vi "Convert Buttons.vi"(7 "POVs":i16[](array[numeric]), 8 "HW_Button Board":bool[](array[boolean]), 9 "HW_Button Board_Axes":dbl[](array[numeric]), 10 "HW_Joystick_Buttons":bool[](array[boolean]), 11 "HW_Joystick_Axes":dbl[](array[numeric])) -> ()   [LabVIEW 2017, in "Controller.lvlib"]
doc: "This VI provides a central place to assign joystick buttons to sepcifc tasks. It aids in the readability of the code and makes it easier to change button assignments."
uses:
  Controller.lvlib
  ENUM_Botton Board.ctl
  ENUM_Logitech Extrem 3D Pro Buttons.ctl
  Global Control Outputs.vi
  ENUM_Logitech GamePad Button List.ctl
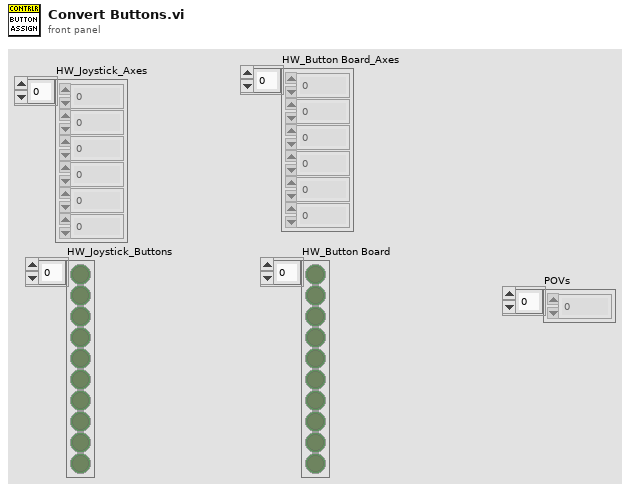
[diagram p1: front panel]
types:
  T1 = typedef "Controller.lvlib/ENUM_Botton Board.ctl" = enum16{"Top Right", "Top Left", "Center Right", "Center Middle", "Center Left", "Bottom Right", "Bottom Middle", "Botton Left"}
  T2 = typedef "Controller.lvlib/ENUM_Logitech GamePad Button List.ctl" = enum16{"Right Pad A-Green", "Right Pad B-Red", "Right Pad X-Blue", "Right Pad Y-Yellow", "Left Trigger LB", "Right Trigger RB", "Center Pad Back", "Center Pad Start", "Left Thumb", "Right Thumb"}
  T3 = typedef "Controller.lvlib/ENUM_Logitech Extrem 3D Pro Buttons.ctl" = enum16{"Trigger (1)", "Thumb (2)", "Upper Top Left (5)", "Upper Lower Left (3)", "Upper Top Right (6)", "Upper Lower Right (4)", "Lower Front Left (7)", "Lower Front Right (8)", "Lower Middle Left (9)", "Lower Middle Right (10)", "Lower Back Left (11)", "Lower (Back Right (12)"}
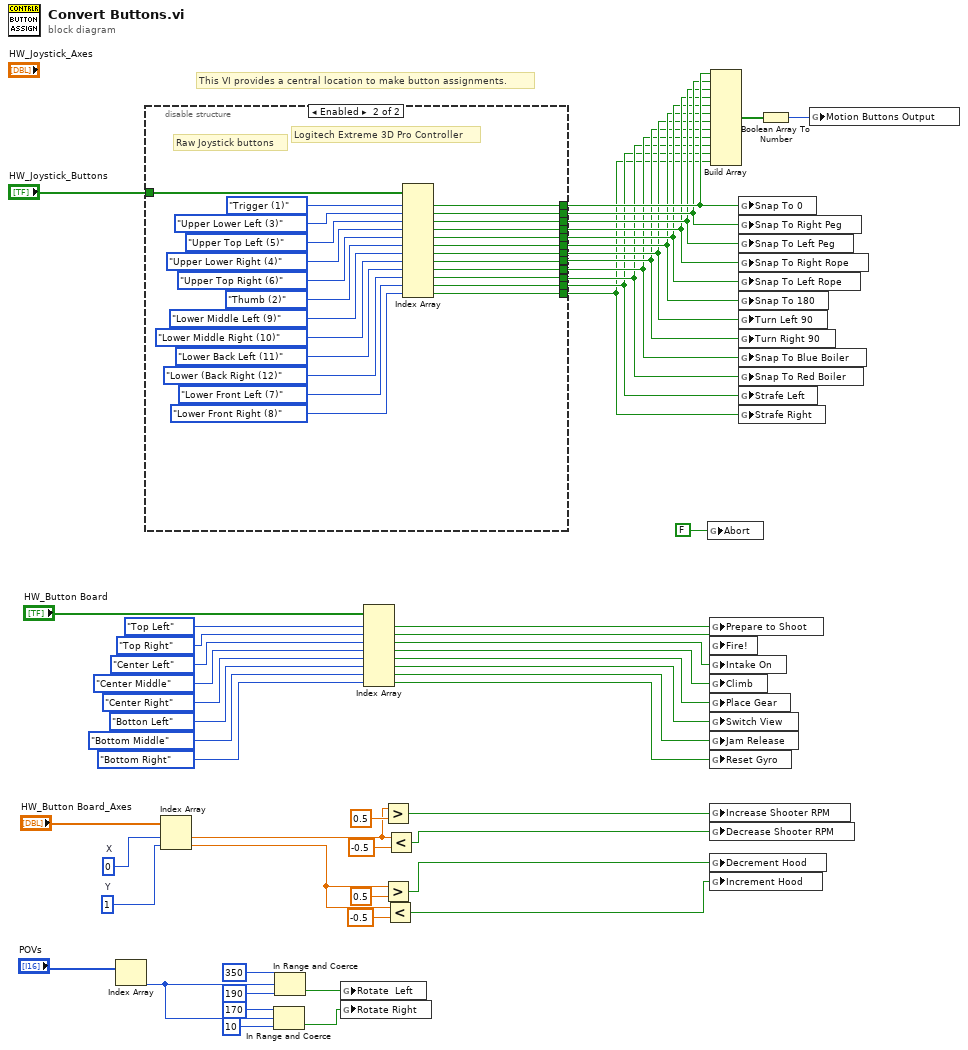
[diagram p0: block diagram]
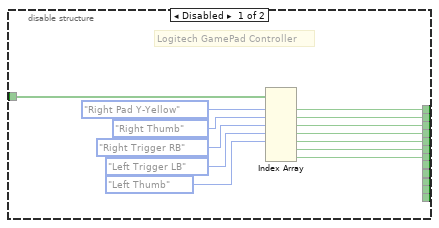
[diagram p2: hidden frame]
diagram:
  w19 = 1  # Y
  w20 = 0  # X
  # "This VI provides a central location to make button assignments."
  n1 = Index Array(array="POVs") -> (element=w7:i16)  [unwired: 1 in]
  n2 = disable-structure shown="Enabled" {
    disable-tunnel: "HW_Joystick_Buttons" -> [w67 w92]
    disable-tunnel: [w65 w87] -> w52
    disable-tunnel: [w61 w86] -> w51
    disable-tunnel: [w60 w85] -> w50
    disable-tunnel: [w59 w84] -> w49
    disable-tunnel: [w57 w82] -> w47
    disable-tunnel: [w56 w81] -> w46
    disable-tunnel: [w55 w83] -> w48
    disable-tunnel: [_ w80] -> w45
    disable-tunnel: [_ w79] -> w44
    disable-tunnel: [_ w78] -> w43
    disable-tunnel: [_ w77] -> w42
    disable-tunnel: [_ w76] -> w41
    frame Disabled {
      # "Logitech GamePad Controller"
      n3 = Index Array(array=w67, index #1=ENUM_Logitech_GamePad_Button_List."Right Pad Y-Yellow" ("Controler Button List"), index #2=ENUM_Logitech_GamePad_Button_List."Right Thumb" ("Controler Button List"), index #3=ENUM_Logitech_GamePad_Button_List."Right Trigger RB" ("Controler Button List"), index #4=ENUM_Logitech_GamePad_Button_List."Left Trigger LB" ("Controler Button List"), index #5=ENUM_Logitech_GamePad_Button_List."Left Thumb" ("Controler Button List")) -> (element #1=w65:bool, element #2=w61:bool, element #3=w60:bool, element #4=w59:bool, element #5=w55:bool, element #6=w57:bool, element #7=w56:bool)  [unwired: 2 in]
    }
    frame Enabled {
      # "Raw Joystick buttons"
      # "Logitech Extreme 3D Pro Controller"
      n4 = Index Array(array=w92, index #1=ENUM_Logitech_Extrem_3D_Pro_Buttons."Trigger (1)" ("Logitech Extreme 3D Pro Buttons"), index #2=ENUM_Logitech_Extrem_3D_Pro_Buttons."Upper Lower Left (3)" ("Logitech Extreme 3D Pro Buttons"), index #3=ENUM_Logitech_Extrem_3D_Pro_Buttons."Upper Top Left (5)" ("Logitech Extreme 3D Pro Buttons"), index #4=ENUM_Logitech_Extrem_3D_Pro_Buttons."Upper Lower Right (4)" ("Logitech Extreme 3D Pro Buttons"), index #5=ENUM_Logitech_Extrem_3D_Pro_Buttons."Upper Top Right (6)" ("Logitech Extreme 3D Pro Buttons"), index #6=ENUM_Logitech_Extrem_3D_Pro_Buttons."Thumb (2)" ("Logitech Extreme 3D Pro Buttons"), index #7=ENUM_Logitech_Extrem_3D_Pro_Buttons."Lower Middle Left (9)" ("Logitech Extreme 3D Pro Buttons"), index #8=ENUM_Logitech_Extrem_3D_Pro_Buttons."Lower Middle Right (10)" ("Logitech Extreme 3D Pro Buttons"), index #9=ENUM_Logitech_Extrem_3D_Pro_Buttons."Lower Back Left (11)" ("Logitech Extreme 3D Pro Buttons"), index #10=ENUM_Logitech_Extrem_3D_Pro_Buttons."Lower (Back Right (12)" ("Logitech Extreme 3D Pro Buttons"), index #11=ENUM_Logitech_Extrem_3D_Pro_Buttons."Lower Front Left (7)" ("Logitech Extreme 3D Pro Buttons"), index #12=ENUM_Logitech_Extrem_3D_Pro_Buttons."Lower Front Right (8)" ("Logitech Extreme 3D Pro Buttons")) -> (element #1=w87:bool, element #2=w86:bool, element #3=w85:bool, element #4=w84:bool, element #5=w83:bool, element #6=w82:bool, element #7=w81:bool, element #8=w80:bool, element #9=w79:bool, element #10=w78:bool, element #11=w77:bool, element #12=w76:bool)
    }
  }
  n5 = Index Array(array="HW_Button Board_Axes", index #1=w20, index #2=w19) -> (element #1=w15:dbl, element #2=w9:dbl)
  n6 = In Range and Coerce(upper limit=i16 170, x=w7, lower limit=i16 10) -> (In Range?=w1:bool)  [unwired: 1 out]
  n7 = In Range and Coerce(upper limit=i16 350, x=w7, lower limit=i16 190) -> (In Range?=w2:bool)  [unwired: 1 out]
  n8 = global write "Global Control Outputs.vi" "Rotate  Left"(w2) -> ()
  n9 = global write "Global Control Outputs.vi" "Rotate Right"(w1) -> ()
  n10 = Index Array(array="HW_Button Board", index #1=ENUM_Botton_Board."Top Left" ("Control Board Buttons"), index #2=ENUM_Botton_Board."Top Right" ("Control Board Buttons"), index #3=ENUM_Botton_Board."Center Left" ("Control Board Buttons"), index #4=ENUM_Botton_Board."Center Middle" ("Control Board Buttons"), index #5=ENUM_Botton_Board."Center Right" ("Control Board Buttons"), index #6=ENUM_Botton_Board."Botton Left" ("Control Board Buttons"), index #7=ENUM_Botton_Board."Bottom Middle" ("Control Board Buttons"), index #8=ENUM_Botton_Board."Bottom Right" ("Control Board Buttons")) -> (element #1=w39:bool, element #2=w30:bool, element #3=w29:bool, element #4=w28:bool, element #5=w27:bool, element #6=w26:bool, element #7=w25:bool, element #8=w24:bool)
  n11 = Greater?(x=w15, y=0.5) -> (0:w17:bool)
  n12 = Greater?(x=w9, y=0.5) -> (0:w12:bool)
  n13 = Less?(x=w9, y=-0.5) -> (x < y?=w13:bool)
  n14 = Less?(x=w15, y=-0.5) -> (x < y?=w14:bool)
  n15 = global write "Global Control Outputs.vi" "Abort"(FALSE) -> ()
  n16 = global write "Global Control Outputs.vi" "Prepare to Shoot"(w39) -> ()
  n17 = global write "Global Control Outputs.vi" "Fire!"(w30) -> ()
  n18 = global write "Global Control Outputs.vi" "Intake On"(w29) -> ()
  n19 = global write "Global Control Outputs.vi" "Climb"(w28) -> ()
  n20 = global write "Global Control Outputs.vi" "Place Gear"(w27) -> ()
  n21 = global write "Global Control Outputs.vi" "Switch View"(w26) -> ()
  n22 = global write "Global Control Outputs.vi" "Jam Release"(w25) -> ()
  n23 = global write "Global Control Outputs.vi" "Reset Gyro"(w24) -> ()
  n24 = global write "Global Control Outputs.vi" "Increase Shooter RPM"(w17) -> ()
  n25 = global write "Global Control Outputs.vi" "Decrease Shooter RPM"(w14) -> ()
  n26 = global write "Global Control Outputs.vi" "Decrement Hood"(w12) -> ()
  n27 = global write "Global Control Outputs.vi" "Increment Hood"(w13) -> ()
  n28 = Build Array(w52, w51, w50, w49, w48, w47, w46, w45, w44, w43, w42, w41) -> (w40:bool[])
  n29 = global write "Global Control Outputs.vi" "Snap To 0"(w52) -> ()
  n30 = global write "Global Control Outputs.vi" "Snap To Right Peg"(w51) -> ()
  n31 = global write "Global Control Outputs.vi" "Snap To Left Peg"(w50) -> ()
  n32 = global write "Global Control Outputs.vi" "Snap To Right Rope"(w49) -> ()
  n33 = global write "Global Control Outputs.vi" "Snap To Left Rope"(w48) -> ()
  n34 = global write "Global Control Outputs.vi" "Snap To 180"(w47) -> ()
  n35 = global write "Global Control Outputs.vi" "Turn Left 90"(w46) -> ()
  n36 = global write "Global Control Outputs.vi" "Turn Right 90"(w45) -> ()
  n37 = global write "Global Control Outputs.vi" "Snap To Blue Boiler"(w44) -> ()
  n38 = global write "Global Control Outputs.vi" "Snap To Red Boiler"(w43) -> ()
  n39 = global write "Global Control Outputs.vi" "Strafe Left"(w42) -> ()
  n40 = global write "Global Control Outputs.vi" "Strafe Right"(w41) -> ()
  n41 = Boolean Array To Number(Boolean array=w40) -> (number=w22:u32)
  n42 = global write "Global Control Outputs.vi" "Motion Buttons Output"(w22) -> ()
